vi "Write to Memory_Core.vi"(0 "data in":T1[](array[typedef]), 9 "input valid":bool, 11 "niUSRP Rx Core v1 FPGA.lvclass":refnum<class "niUSRP Sync v1 FPGA.lvclass">, 12 "ready for output":bool) -> (14 "ready for input":bool, 15 "niUSRP Rx Core v1 FPGA.lvclass 2":refnum<class "niUSRP Sync v1 FPGA.lvclass">)   [LabVIEW 2025, in "niUSRP Sync v1 FPGA.lvclass"]
uses:
  niUSRP Sync v1 FPGA.lvclass
  niUSRP Sync v1 FPGA.lvclass/niUSRP Sync v1 FPGA.ctl
  <instrlib>/_niInstr/DSP/v1/FPGA/niInstr DSP v1 FPGA.lvlib
  <instrlib>/_niInstr/Basic Elements/v1/FPGA/niInstr Basic Elements v1 FPGA.lvlib
  <vilib>/rvi/DataTransferAndStorage/Container/XNode/niFpgaContainer.xnode
  <instrlib>/_niInstr/Basic Elements/v1/FPGA/Private/Write U32 FIFO.vi
  <instrlib>/_niInstr/DSP/v1/FPGA/Public/Sub VIs/Data Conversion/IQ to U32 - N spc - S18.1.vi
  <vilib>/rvi/DataTransferAndStorage/Register/Emulation/niFpgaRegisterEmulationRefIn.vi
  <instrlib>/_niInstr/DSP/v1/Shared/Public/IQ Data.ctl
  <instrlib>/_niInstr/DSP/v1/Shared/niInstr DSP v1 Shared.lvlib
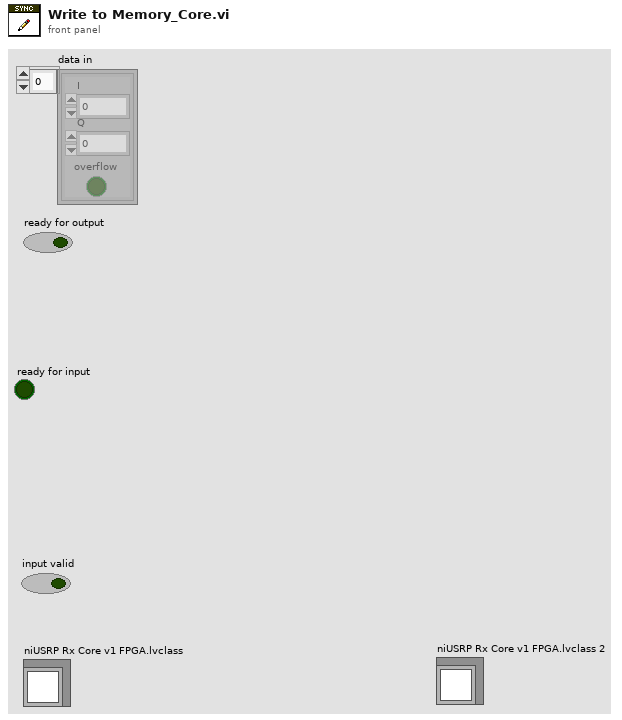
[diagram p1: front panel]
types:
  T1 = typedef "niInstr DSP v1 Shared.lvlib/IQ Data.ctl" = cluster{"I":fxp<+/-,18,1>, "Q":fxp<+/-,18,1>, "overflow":bool}
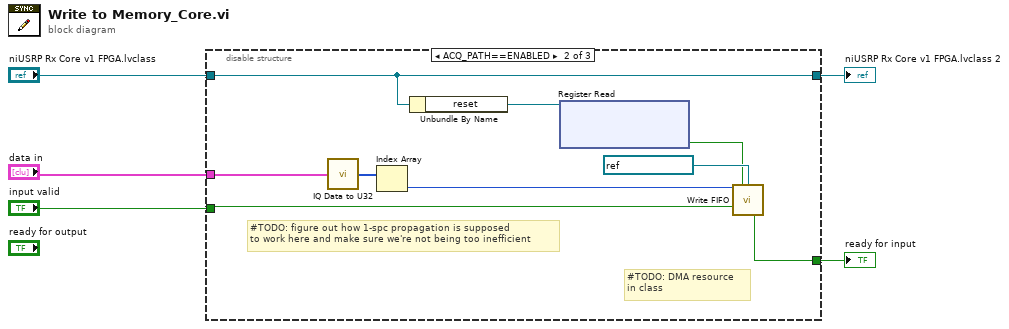
[diagram p0: block diagram]
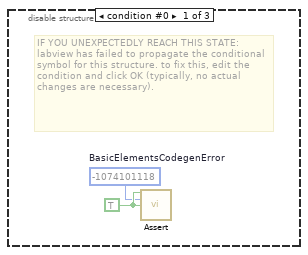
[diagram p2: hidden frame]
diagram:
  n1 = disable-structure shown="ACQ_PATH==ENABLED" {
    disable-tunnel: "data in" -> [_ w10 _]
    disable-tunnel: "input valid" -> [_ w12 _]
    disable-tunnel: "niUSRP Rx Core v1 FPGA.lvclass" -> [_ w13 _]
    disable-tunnel: [_ w13 _] -> w2
    disable-tunnel: [_ w11 _] -> w1
    frame condition #0 {
      w7 = TRUE ("assert")
      w6 = -1074101118  # BasicElementsCodegenError
      # "IF YOU UNEXPECTEDLY REACH THIS STATE:\nlabview has failed to propagate the conditional symbol for this structure. to fix this, edit the condition and click OK (typically, no actual changes are necessary)."
      n2 = call <instrlib>:"Assert.vi"("assert"=w7, "error code"=w6, "enable show error"=w7) -> ()  [unwired: 13 in]
    }
    frame condition #1 (active) {
      # "#TODO: DMA resource\nin class"
      # "#TODO: figure out how 1-spc propagation is supposed\nto work here and make sure we're not being too inefficient"
      n3 = call-poly <instrlib>:"IQ Data to U32.vi"("IQ data"=w10) -> ("U32 data"=w9:u32[])  [unwired: 13 in, 1 out]
      n4 = Index Array(array=w9) -> (element=w8:u32)  [unwired: 1 in]
      n5 = Unbundle By Name(w13) -> ("reset"=w16:refnum<k21>)
      n6 = xnode ("Register Read")("Register In"=w16) -> ("Data"=w14:bool)  [unwired: 1 out]
      n7 = call-poly <instrlib>:"Write FIFO.vi"("input data"=w8, "reset"=w14, "fifo"=refnum<k21> "Rx Stream 0" ("FIFO 0"), "input valid"=w12) -> ("ready for input"=w11:bool)  [unwired: 11 in]
    }
    frame condition #2 {
    }
  }
  "niUSRP Rx Core v1 FPGA.lvclass 2" <- w2
  "ready for input" <- w1
